vi "Full_Sweep_ODFT_iHV.vi"(10 "Ext_HV":dbl=38.0 format="%#_13g", 11 "Semiconductor Module Context":T1) -> (0 "error out":errorcluster)   [LabVIEW 2013]
uses:
  <vilib>/NI_TestStand_SemiconductorModule/NI_TestStand_Semiconductor_Module.lvlibp/PinMap/General/SemiconductorModuleContext.ctl
  <instrlib>/niHSDIO/niHSDIO.llb/niHSDIO_ctl Trigger Script - trigID Values (Ring).ctl
  <vilib>/NI_TestStand_SemiconductorModule/NI_TestStand_Semiconductor_Module.lvlibp/PinMap/DC Power/PinsToNIDCPowerSessions.vi
  <vilib>/NI_TestStand_SemiconductorModule/NI_TestStand_Semiconductor_Module.lvlibp/PinMap/Deprecated/PublishDataDoubleMultiplePinsMultipleInstruments.vi
  <vilib>/NI_TestStand_SemiconductorModule/NI_TestStand_Semiconductor_Module.lvlibp
panel:
  out "current measurements":dbl[][][](array[numeric])
  in  "Pins":string[](array[string])=["HV"]
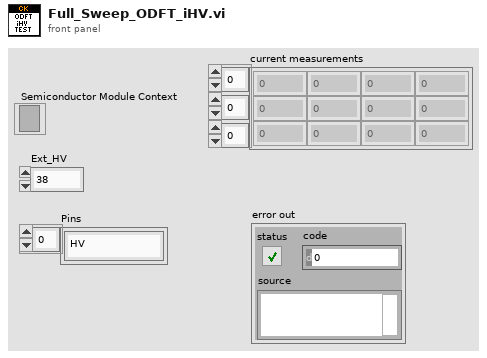
[diagram p1: front panel]
types:
  T1 = typedef "NI_TestStand_Semiconductor_Module.lvlibp/SemiconductorModuleContext.ctl" = refnum<k7>
  T2 = typedef "niHSDIO_ctl Trigger Script - trigID Values (Ring).ctl" = string
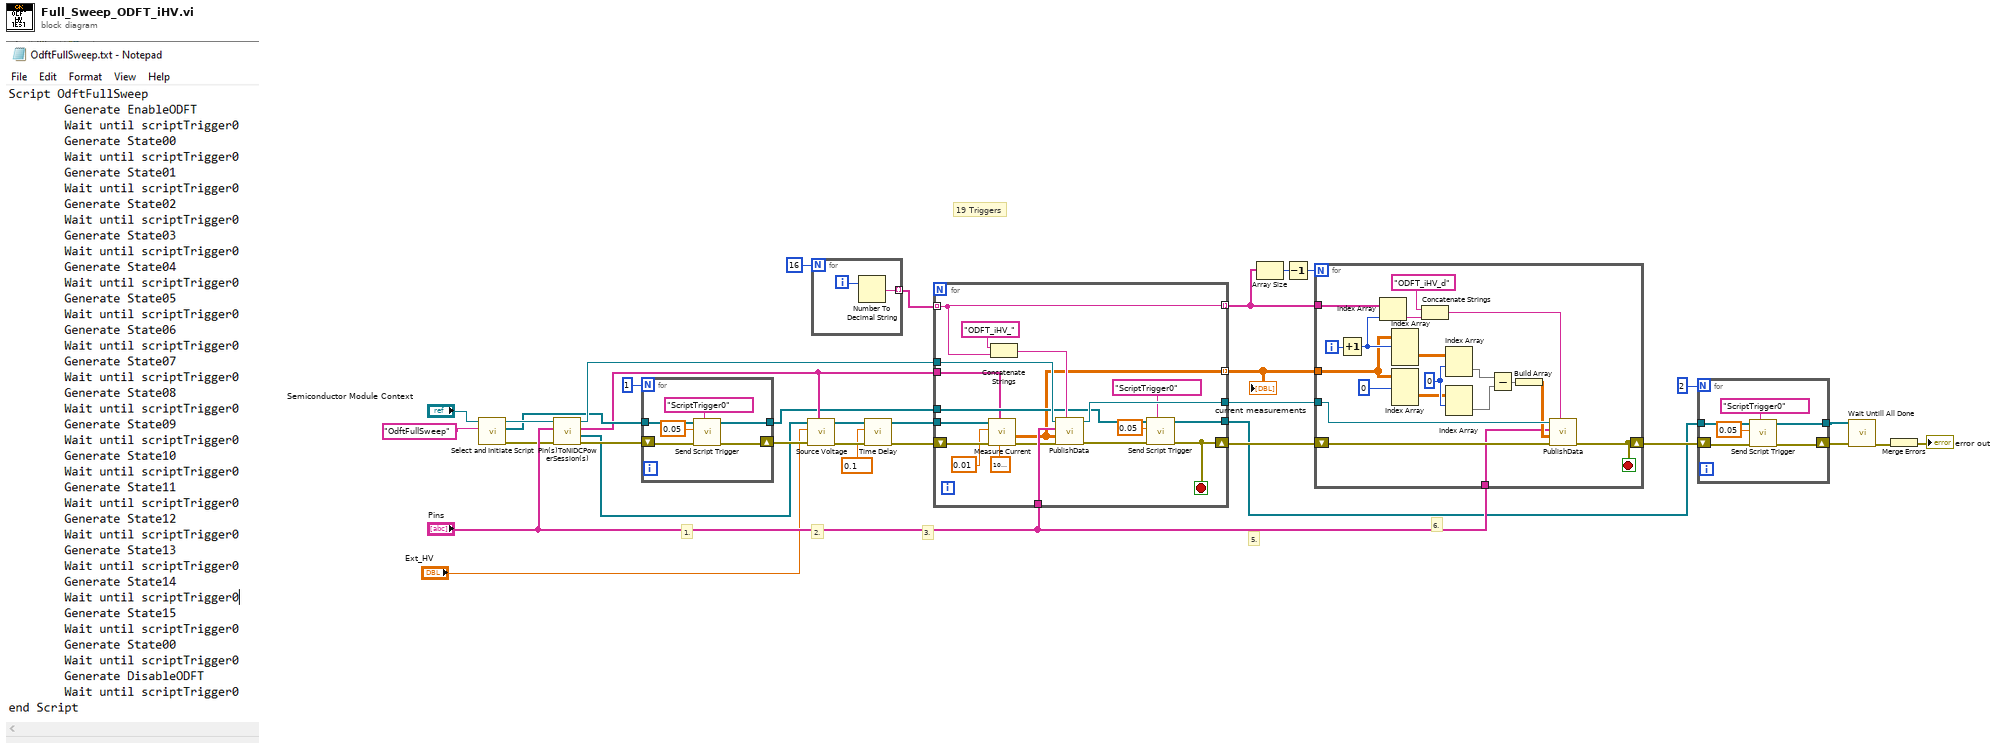
[diagram p0: block diagram]
diagram:
  # "19 Triggers"
  # "3."
  # "6."
  # "5."
  # "2."
  # "1."
  n1 = call "Select and Initiate Script.vi"("script name"="OdftFullSweep", "Semiconductor Module Context"="Semiconductor Module Context") -> ("error out"=w17:errorcluster, "HSDIO GEN Sessions Out"=w18:refnum<k15>[], "Semiconductor Module Context Out"=w19:T1)  [unwired: 7 in]
  n2 = call-poly <vilib>:"Pin(s)ToNIDCPowerSession(s).vi"("error in (no error)"=w17, "Pins"="Pins", "Semiconductor Module Context"=w19) -> ("error out"=w32:errorcluster, "Instrument Sessions"=w16:refnum<k15>[], "Channel Lists"=w15:string[], "Semiconductor Module Context Out"=w21:T1)  [unwired: 4 in, 1 out]
  n3 = for {
    N: 1 -> [_]
    shift-right: [w37] -> w30
    shift-left: w32 -> [w38]
    tunnel: w18 -> [w36]
    tunnel: [w35] -> w13
    n4 = call "Send Script Trigger.vi"("trigger id (script trigger 0)"=T2 "ScriptTrigger0", "error in (no error)"=w38, "Delay Time (s)"=0.05, "HSDIO Sessions In"=w36) -> ("error out"=w37:errorcluster, "HSDIO Sessions Out"=w35:refnum<k15>[])  [unwired: 6 in]
  }
  n5 = call "Source Voltage.vi"("Channel Lists"=w15, "error in (no error)"=w30, "voltage level"="Ext_HV", "Instrument Sessions In"=w16) -> ("error out"=w11:errorcluster, "Instrument Sessions Out"=w29:refnum<k15>[])  [unwired: 4 in, 2 out]
  n6 = for {
    N: 16 -> [_]
    tunnel: [w40] -> w1 mode=indexing
    i -> [w41]
    n7 = Number To Decimal String(number=w41) -> (decimal integer string=w40:string)  [unwired: 1 in]
  }
  n8 = call "Time Delay"("error in (no error)"=w11, "Delay Time (s)"=0.1) -> ("error out"=w10:errorcluster)  [unwired: 9 in]
  n9 = for {
    tunnel: w1 -> [w57] mode=indexing
    tunnel: w29 -> [w47]
    tunnel: w21 -> [w58]
    shift-right: [w51] -> w28
    shift-left: w10 -> [w49]
    tunnel: [w57] -> w26 mode=indexing
    tunnel: "Pins" -> [w56]
    tunnel: w13 -> [w52]
    tunnel: [w55] -> w23
    tunnel: w15 -> [w46]
    tunnel: [w50] -> w12 mode=indexing
    tunnel: [w43] -> w6
    stop <- w51 stop-if-true
    n10 = call "Measure Current.vi"("Result Multiplier"=1000000.0, "Channel Lists"=w46, "error in (no error)"=w49, "Delay Time (s)"=0.01, "DCPower Sessions In"=w47) -> ("error out"=w48:errorcluster, "current measurements"=w50:dbl[][])  [unwired: 4 in, 1 out]
    n11 = Concatenate Strings("ODFT_iHV_", w57) -> (w60:string)
    n12 = call-poly <vilib>:"PublishData.vi"("Measurement Id"=w60, "error in (no error)"=w48, "Data In"=w50, "Pins"=w56, "Semiconductor Module Context"=w58) -> ("error out"=w54:errorcluster, "Semiconductor Module Context Out"=w55:T1)  [unwired: 5 in]
    n13 = call "Send Script Trigger.vi"("trigger id (script trigger 0)"=T2 "ScriptTrigger0", "error in (no error)"=w54, "Delay Time (s)"=0.05, "HSDIO Sessions In"=w52) -> ("error out"=w51:errorcluster, "HSDIO Sessions Out"=w43:refnum<k15>[])  [unwired: 6 in]
  }
  "current measurements" <- w12
  n14 = Array Size(array=w26) -> (size(s)=w25:i32)
  n15 = Decrement(x=w25) -> (x-1=w24:i32)
  n16 = for {
    N: w24 -> [_]
    tunnel: w26 -> [w76]
    shift-right: [w69] -> w7
    shift-left: w28 -> [w74]
    tunnel: "Pins" -> [w61]
    tunnel: w23 -> [w70]
    tunnel: w12 -> [w68]
    i -> [w77]
    stop <- w69 stop-if-true
    w71 = 0 ("index (page)")
    n17 = Increment(x=w77) -> (x+1=w72:i32)
    n18 = Index Array(array=w76, index=w72) -> (element=w75:string)
    n19 = Index Array(array=w68, index (dim 0)=w72) -> (element=w67:dbl[][])  [unwired: 2 in]
    n20 = Index Array(array=w68, index (dim 0)=0 ("index (page)")) -> (element=w66:dbl[][])  [unwired: 2 in]
    n21 = Concatenate Strings("ODFT_iHV_d", w75) -> (w78:string)
    n22 = Index Array(array=w67, index (row)=w71) -> (element=w64:dbl[])  [unwired: 1 in]
    n23 = Index Array(array=w66, index (row)=w71) -> (element=w65:dbl[])  [unwired: 1 in]
    n24 = Subtract(x=w64, y=w65) -> (x-y=w63:dbl[])
    n25 = Build Array(w63) -> (w62:dbl[][])
    n26 = call-poly <vilib>:"PublishData.vi"("Measurement Id"=w78, "error in (no error)"=w74, "Data In"=w62, "Pins"=w61, "Semiconductor Module Context"=w70) -> ("error out"=w69:errorcluster)  [unwired: 5 in, 1 out]
  }
  n27 = for {
    N: 2 -> [_]
    shift-right: [w83] -> w4
    shift-left: w7 -> [w84]
    tunnel: w6 -> [w82]
    tunnel: [w81] -> w5
    n28 = call "Send Script Trigger.vi"("trigger id (script trigger 0)"=T2 "ScriptTrigger0", "error in (no error)"=w84, "Delay Time (s)"=0.05, "HSDIO Sessions In"=w82) -> ("error out"=w83:errorcluster, "HSDIO Sessions Out"=w81:refnum<k15>[])  [unwired: 6 in]
  }
  n29 = call "Wait Untill All Done.vi"("error in (no error)"=w4, "HSDIO Sessions In"=w5) -> ("error out"=w14:errorcluster)  [unwired: 8 in, 1 out]
  n30 = Merge Errors(w14) -> (→"error out":errorcluster)
